vi "Weapon Probe.vi"(11 "Laser out":refnum<class "Laser.lvclass">) -> (2 "Value String":string, 3 "Boolean":bool)   [LabVIEW 2021, in "Weapon.lvclass"]
uses:
  Weapon/Weapon.lvclass
  Weapons/Laser/Laser.lvclass
  C:/dev/LabVIEW/LabMelee/Source/Application Specific/Element/Element.lvclass
  Element/Element.lvclass/Element.ctl
  Motion/Motion.lvclass/Motion.ctl
  Vector 2D/Vector 2D.lvclass/Vector 2D.ctl
  Element/Element.lvclass
  Vector 2D/Vector 2D.lvclass
panel:
  out "y":sgl
  out "x":sgl
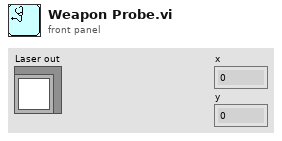
[diagram p1: front panel]
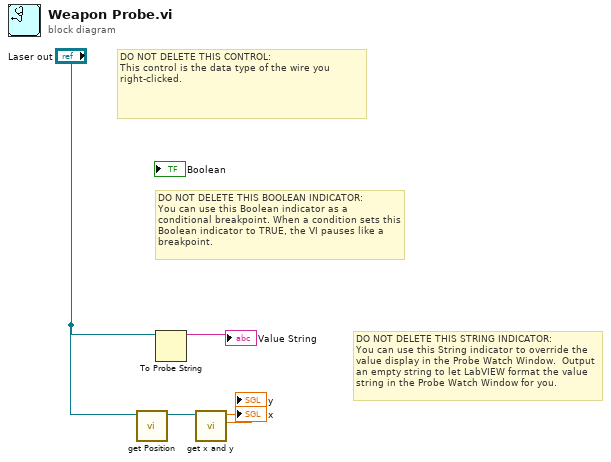
[diagram p0: block diagram]
diagram:
  # "DO NOT DELETE THIS STRING INDICATOR: \nYou can use this String indicator to override the value display in the Probe Watch Window.  Output an empty string to let LabVIEW format the value string in the Probe Watch Window for you."
  # "DO NOT DELETE THIS BOOLEAN INDICATOR: \nYou can use this Boolean indicator as a conditional breakpoint. When a condition sets this Boolean indicator to TRUE, the VI pauses like a breakpoint."
  # "DO NOT DELETE THIS CONTROL: \nThis control is the data type of the wire you right-clicked."
  n1 = call "get Position.vi"("Element in"="Laser out") -> ("Position"=w3:refnum<class "Vector 2D.lvclass">)  [unwired: 10 in]
  n2 = To Probe String(7:"Laser out") -> (3:→"Value String":string)  [unwired: 2 in, 1 out]
  n3 = call "get x and y.vi"("Vector 2D in"=w3) -> ("y"=→"y":sgl, "x"=→"x":sgl)  [unwired: 9 in]
